vi "labviewParse.vi"() -> ()   [LabVIEW 2021]
uses:
  Program Files (x86)/National Instruments/LabVIEW 2021/examples/Connectivity/Python/support/PythonVersionsEnum.ctl
panel:
  out "error out":errorcluster
  in  "error in (no error)":errorcluster
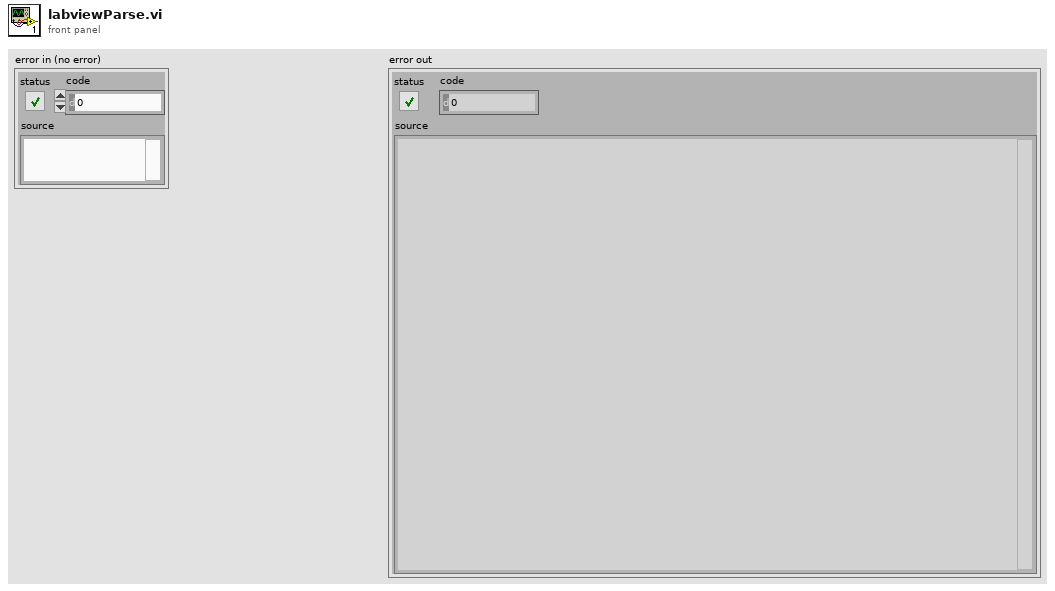
[diagram p1: front panel]
types:
  T1 = typedef "PythonVersionsEnum.ctl" = enum16{"3.6", "3.7", "3.8", "3.9"}
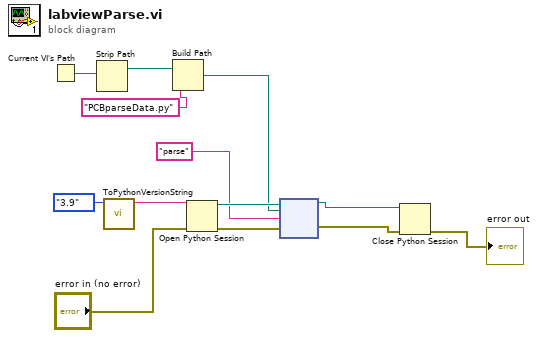
[diagram p0: block diagram]
diagram:
  n1 = Current VI's Path() -> (path=w2:path)
  n2 = Strip Path(path=w2) -> (stripped path=w8:path)  [unwired: 1 out]
  n3 = call "ToPythonVersionString.vi"("python version"=PythonVersionsEnum."3.9") -> ("python version string"=w12:string)  [unwired: 10 in]
  n4 = Build Path(base path=w8, name or relative path="PCBparseData.py") -> (appended path=w6:path)
  n5 = Open Python Session(python version=w12, 3:"error in (no error)") -> (session out=w10:refnum<k35>, error out=w9:errorcluster)  [unwired: 1 in]
  n6 = node(w10, w6, "parse" ("function name"), w9) -> (w5:refnum<k35>, w4:errorcluster)  [unwired: 2 in, 2 out]
  n7 = Close Python Session(session in=w5, error in=w4) -> (11:→"error out":errorcluster)
